vi "Timing.vi"(8 "error in":errorcluster) -> (0 "error out":errorcluster)   [LabVIEW 2012, in "Spinner.xctl"]
uses:
  Spinner.xctl
  Attrs.ctl
  Command.ctl
panel:
  out "delay":u32
  out "stop?":bool
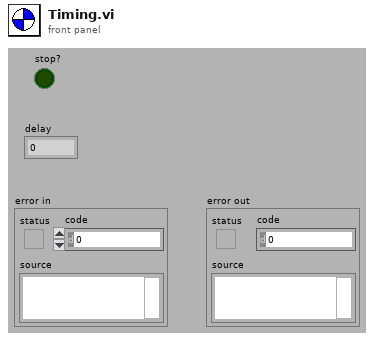
[diagram p1: front panel]
types:
  T1 = typedef "Spinner.xctl/Attrs.ctl" = cluster{"Owner ref":refnum<vi>, "Pic ref":refnum<vi>, "Step len":dbl, "Imgs":picture[], "Current phase":dbl}
  T2 = typedef "Spinner.xctl/Command.ctl" = enum16{"Add Control", "Remove Control", "Update Imgs", "Update Speed", "Refresh"}
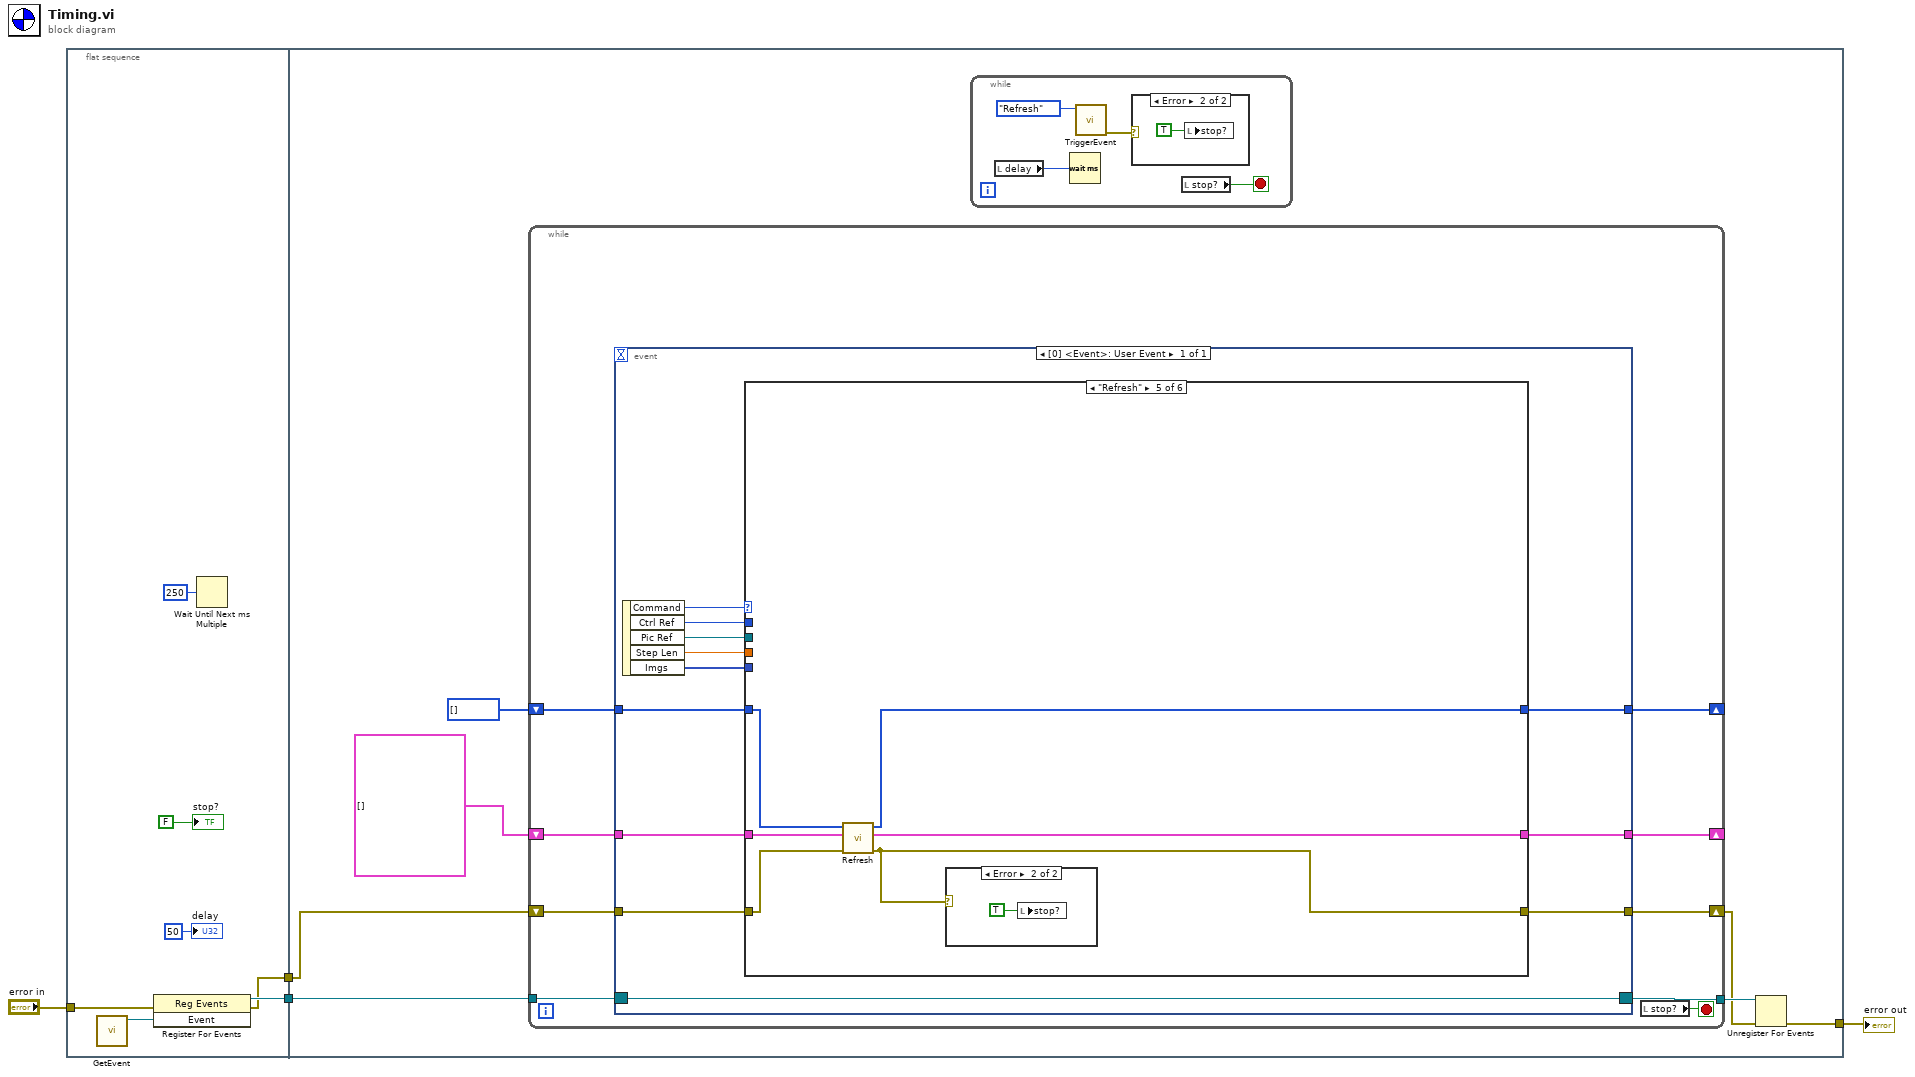
[diagram p0: block diagram]
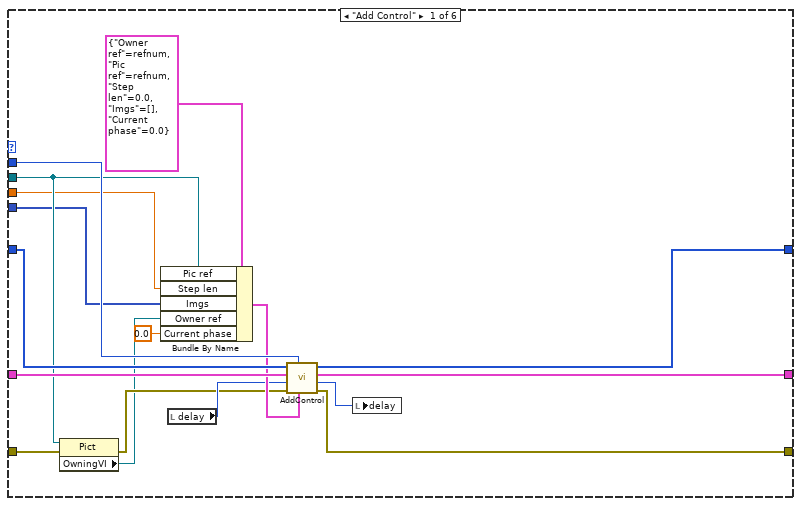
[diagram p3: hidden frame]
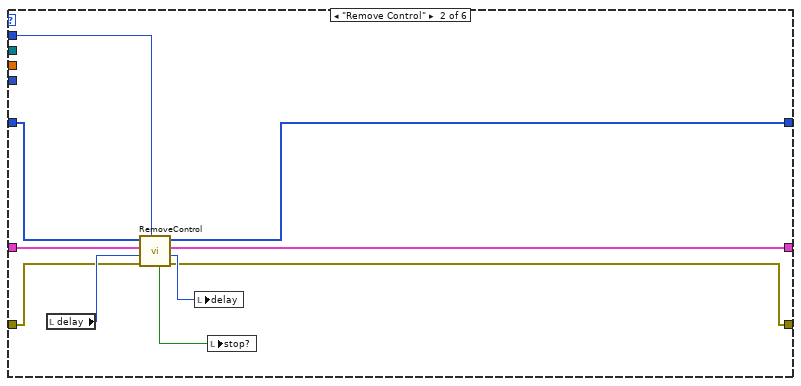
[diagram p4: hidden frame]
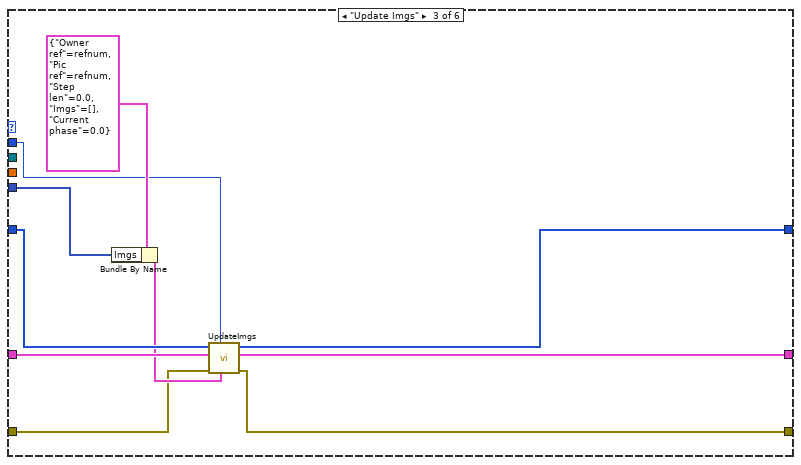
[diagram p5: hidden frame]
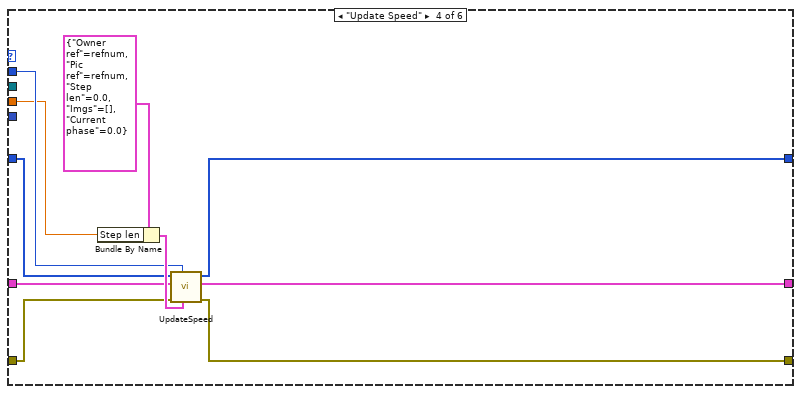
[diagram p6: hidden frame]
diagram:
  n1 = flat-sequence {
    tunnel: [w6] -> w4
    tunnel: [w5] -> w2
    tunnel: "error in" -> [w8]
    tunnel: w4 -> [w15]
    tunnel: w2 -> [w14]
    tunnel: [w12] -> w1
    frame #0 {
      n2 = call "GetEvent.vi"() -> ("Event"=w9:refnum<user-event>)  [unwired: 10 in, 1 out]
      n3 = register-events(error in=w8, w9) -> (reference out=w6:refnum<event-registration>, error out=w5:errorcluster)  [unwired: 1 in]
      n4 = Wait Until Next ms Multiple(millisecond multiple=u32 250) -> ()  [unwired: 1 out]
      "stop?" <- FALSE ("stop?")
      "delay" <- u32 50 ("Delay")
    }
    frame #1 {
      n5 = while {
        shift-right: [w31] -> _
        shift-left: u32[] [] -> [w32]
        tunnel: [w30] -> w17
        shift-right: [w27] -> _
        shift-left: T1[] [] -> [w28]
        tunnel: w15 -> [w26]
        shift-right: [w24] -> w13
        shift-left: w14 -> [w25]
        stop <- w29 stop-if-true
        n6 = event shown="[0] <Event>: User Event" {
          selector: w26 -> [w39]
          dyn-events: [w39] -> w30
          timeout: _ -> [_]
          tunnel: w32 -> [w42]
          tunnel: [w41] -> w31
          tunnel: w28 -> [w36]
          tunnel: [w35] -> w27
          tunnel: w25 -> [w34]
          tunnel: [w33] -> w24
          event User Event {
            n7 = event-data() -> ("Command"=w44:T2, "Ctrl Ref"=w40:u32, "Pic Ref"=w43:refnum<vi>, "Step Len"=w38:dbl, "Imgs"=w37:picture[])  [unwired: 1 in]
            n8 = case shown="\"Refresh\"" w44 {
              tunnel: w43 -> [w49 _ _ _ _ _]
              tunnel: w42 -> [w60 w70 w78 w87 w97 w101]
              tunnel: [w57 w67 w72 w84 w94 w101] -> w41
              tunnel: w40 -> [w59 w71 w79 w89 _ _]
              tunnel: w38 -> [w46 _ _ w88 _ _]
              tunnel: w37 -> [w45 _ w80 _ _ _]
              tunnel: w36 -> [w58 w69 w77 w86 w96 w100]
              tunnel: [w56 w66 w73 w83 w93 w100] -> w35
              tunnel: w34 -> [w52 w63 w75 w85 w95 w99]
              tunnel: [w50 w62 w74 w82 w92 w99] -> w33
              frame "Add Control" {
                n9 = property class="Pict"(reference=w49, error in=w52) -> (error out=w51:errorcluster, "OwningVI"=w47:refnum<vi>)  [unwired: 1 out]
                n10 = Bundle By Name(cluster=T1 {"Owner ref"=refnum, "Pic ref"=refnum, "Step len"=0.0, "Imgs"=[], "Current phase"=0.0} ("Attrs"), "Pic ref"=w49, "Step len"=w46, "Imgs"=w45, "Owner ref"=w47, "Current phase"=0.0) -> (w55:T1)
                n11 = local read "delay"() -> (w54:u32)
                n12 = call "AddControl.vi"("Attrs in"=w55, "Ctrl in"=w59, "error in"=w51, "delay in"=w54, "Attrs array in"=w58, "Ctrl array in"=w60) -> ("error out"=w50:errorcluster, "delay out"=w53:u32, "Attrs array out"=w56:T1[], "Ctrl array out"=w57:u32[])  [unwired: 2 in]
                n13 = local write "delay"(w53) -> ()
              }
              frame "Remove Control" {
                n14 = local read "delay"() -> (w68:u32)
                n15 = call "RemoveControl.vi"("Ctrl in"=w71, "error in"=w63, "delay in"=w68, "Attrs array in"=w69, "Ctrl array in"=w70) -> ("error out"=w62:errorcluster, "delay out"=w64:u32, "Attrs array out"=w66:T1[], "Ctrl array out"=w67:u32[], "stop?"=w65:bool)  [unwired: 2 in]
                n16 = local write "delay"(w64) -> ()
                n17 = local write "stop?"(w65) -> ()
              }
              frame "Update Imgs" {
                n18 = Bundle By Name(cluster=T1 {"Owner ref"=refnum, "Pic ref"=refnum, "Step len"=0.0, "Imgs"=[], "Current phase"=0.0} ("Attrs"), "Imgs"=w80) -> (w76:T1)
                n19 = call "UpdateImgs.vi"("Attrs in"=w76, "Ctrl in"=w79, "error in"=w75, "Attrs array in"=w77, "Ctrl array in"=w78) -> ("error out"=w74:errorcluster, "Attrs array out"=w73:T1[], "Ctrl array out"=w72:u32[])  [unwired: 4 in]
              }
              frame "Update Speed" {
                n20 = Bundle By Name(cluster=T1 {"Owner ref"=refnum, "Pic ref"=refnum, "Step len"=0.0, "Imgs"=[], "Current phase"=0.0} ("Attrs"), "Step len"=w88) -> (w90:T1)
                n21 = call "UpdateSpeed.vi"("Attrs in"=w90, "Ctrl in"=w89, "error in"=w85, "Attrs array in"=w86, "Ctrl array in"=w87) -> ("error out"=w82:errorcluster, "Attrs array out"=w83:T1[], "Ctrl array out"=w84:u32[])  [unwired: 4 in]
              }
              frame "Refresh" {
                n22 = call "Refresh.vi"("error in"=w95, "Attrs array in"=w96, "Ctrl array in"=w97) -> ("error out"=w92:errorcluster, "Attrs array out"=w93:T1[], "Ctrl array out"=w94:u32[])  [unwired: 6 in]
                n23 = case shown="Error" w92 {
                  frame No Error {
                  }
                  frame Error {
                    n24 = local write "stop?"(TRUE ("stop?")) -> ()
                  }
                }
              }
              frame Default {
              }
            }
          }
        }
        n25 = local read "stop?"() -> (w29:bool)
      }
      n26 = while {
        stop <- w22 stop-if-true
        n27 = local read "delay"() -> (w21:u32)
        n28 = Wait (ms)(milliseconds to wait=w21) -> ()  [unwired: 1 out]
        n29 = call "TriggerEvent.vi"("Command"=Command."Refresh") -> ("error out"=w20:errorcluster)  [unwired: 10 in]
        n30 = case shown="Error" w20 {
          frame No Error {
          }
          frame Error {
            n31 = local write "stop?"(TRUE ("stop?")) -> ()
          }
        }
        n32 = local read "stop?"() -> (w22:bool)
      }
      n33 = Unregister For Events(event registration refnum=w17, error in=w13) -> (error out=w12:errorcluster)
    }
  }
  "error out" <- w1
